vi "Item Selection VIG - Originale.vi"(4 "Defer Front Panel (T)":bool, 6 "Shift":bool, 7 "Method (Read Selection)":T1, 8 "error in (no error)":errorcluster, 9 "New Selected Row":i32, 10 "Selection":bool[](array[boolean]), 11 "Listbox or Tree":refnum<vi>) -> (0 "error out":errorcluster, 2 "Tags":string[](array[string]), 3 "Selection":bool[](array[boolean]))   [LabVIEW 2020]
doc: "This is a global VI that maintains the state of <B>Listbox</B> passed in. The first this this is called it should have the <B>Method</B> set to Force Selection which sets the symbols of the contol based on <B>Selection</B>. This VI can then be called to select all, select none, or invert the selection of that control. This VI can also handle the mouse down event on the control, which will set or clear the selection of items based on the <B>New Selected Row</B>, and if the <B>Shift</B> key was being held. The default method will return the <B>Selected Items</B> for that control.\n\nBy default this VI will <B>Defer Front Panel</B> of the front panel of the owning VI and undefer after the selection has finished.\n-------------\nBrian Hoover (hooovahh)"
uses:
  Selection Global Method.ctl
  <userlib>/_OpenG.lib/array/array.llb/Conditional Auto-Indexing Tunnel (String)__ogtk.vi
  <userlib>/_OpenG.lib/array/array.llb/Search 1D Array (Boolean)__ogtk.vi
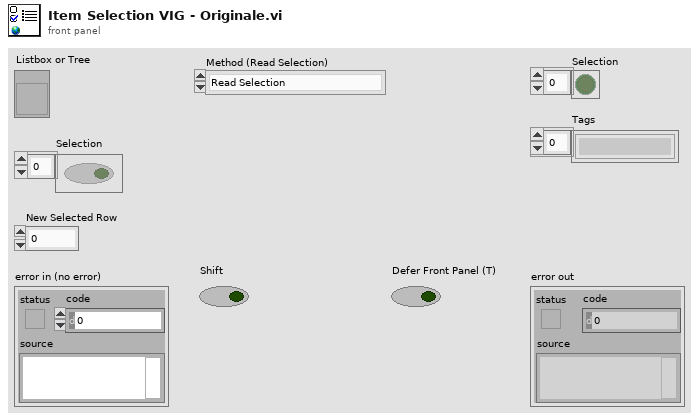
[diagram p1: front panel]
types:
  T1 = typedef "Selection Global Method.ctl" = enum16{"Read Selection", "Force Selection", "Mouse Down Event", "Select All", "Select None", "Invert Selection", "Read Selection and Tags"}
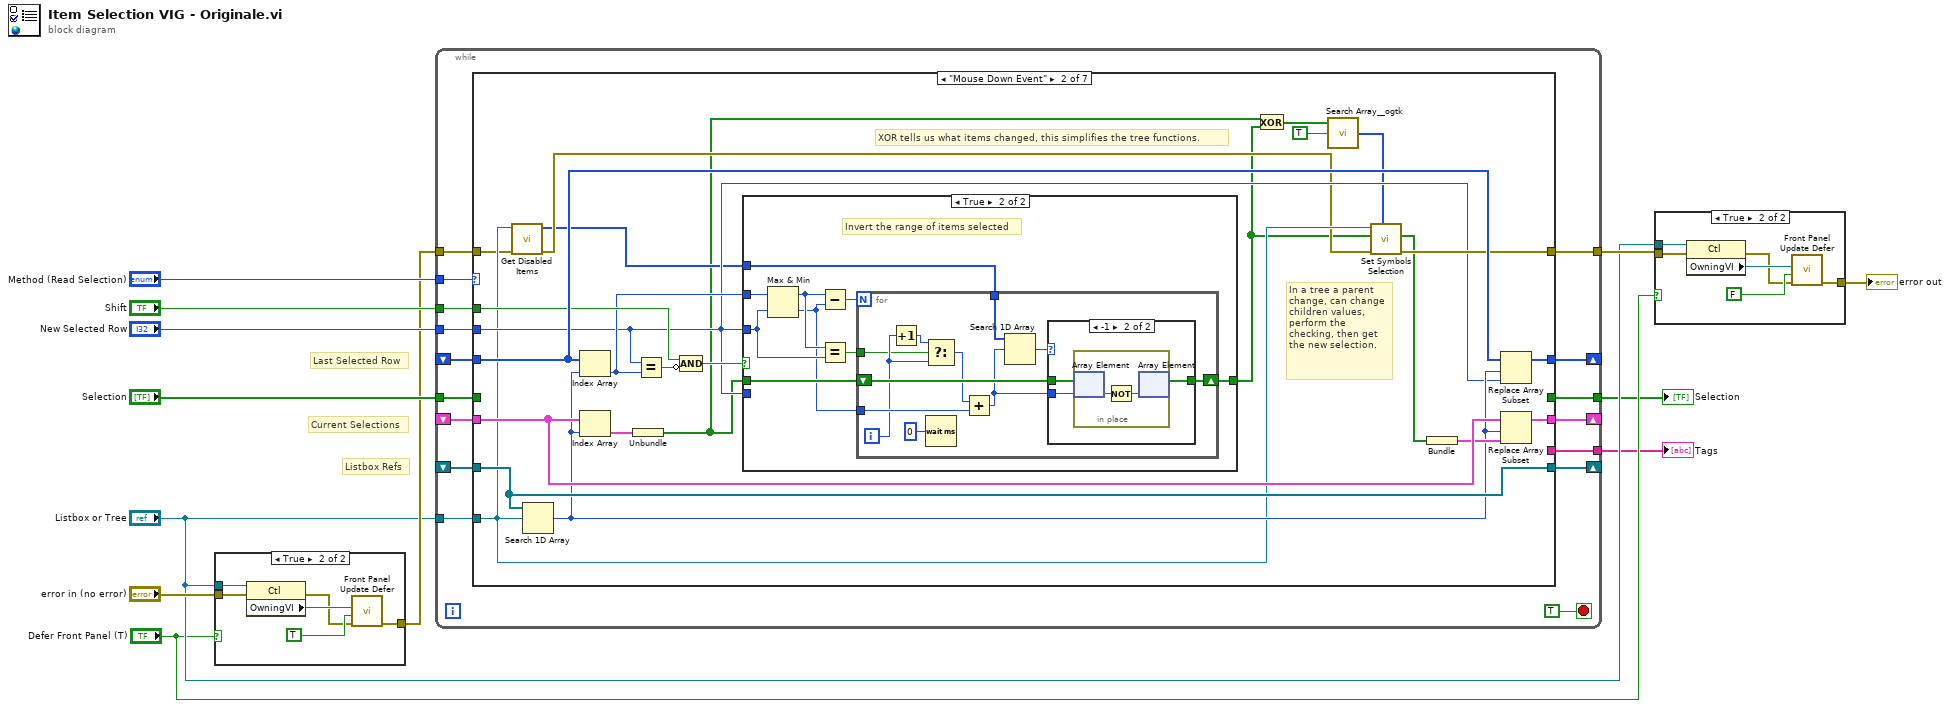
[diagram p0: block diagram]
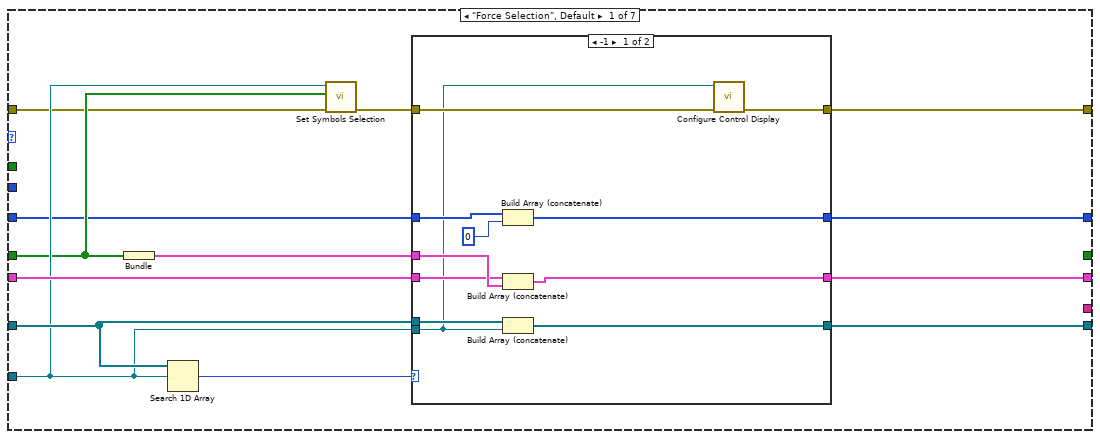
[diagram p4: hidden frame]
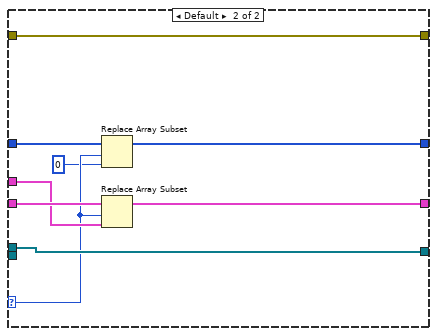
[diagram p5: hidden frame]
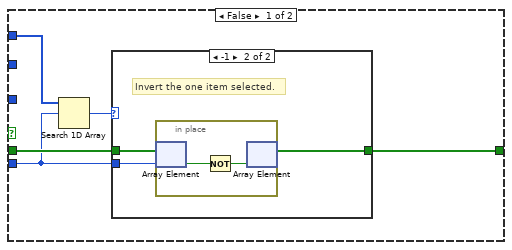
[diagram p6: hidden frame]
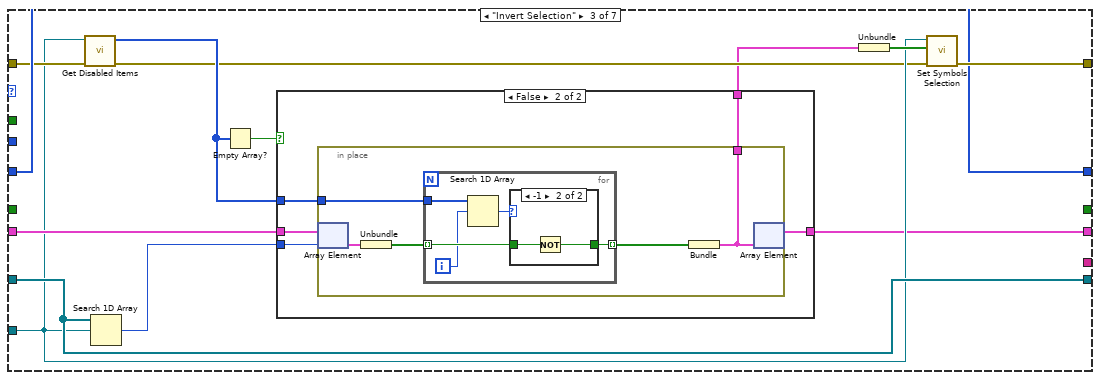
[diagram p9: hidden frame]
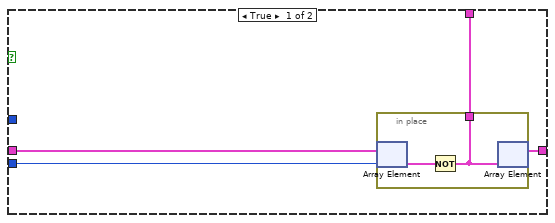
[diagram p10: hidden frame]
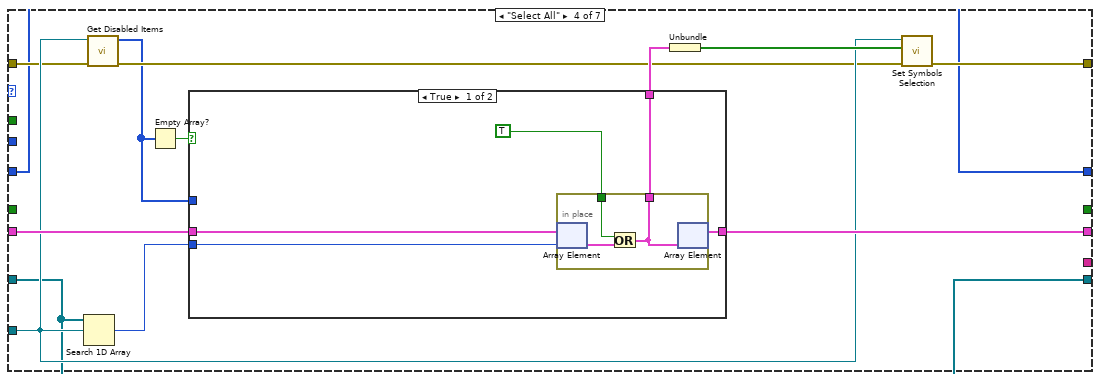
[diagram p12: hidden frame]
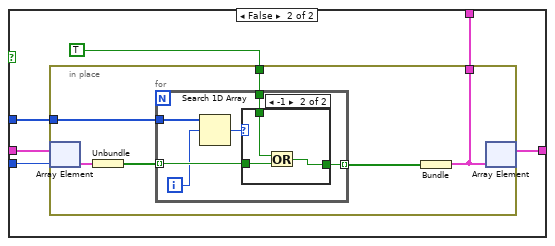
[diagram p13: hidden frame]
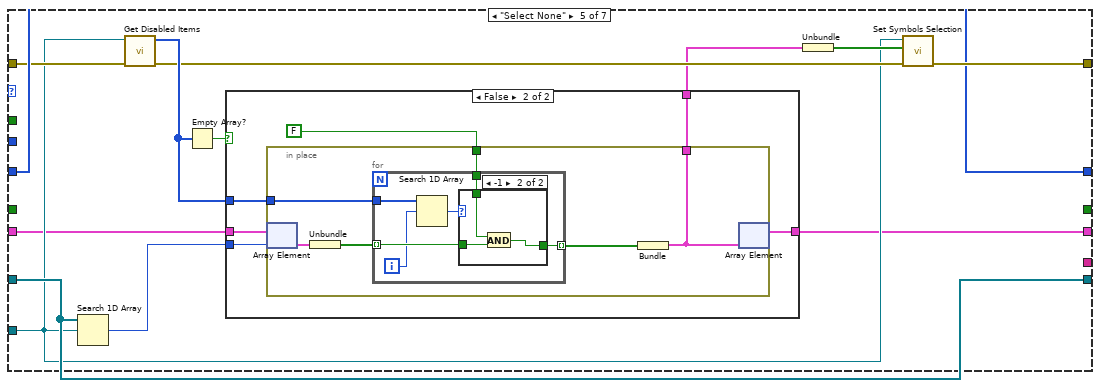
[diagram p15: hidden frame]
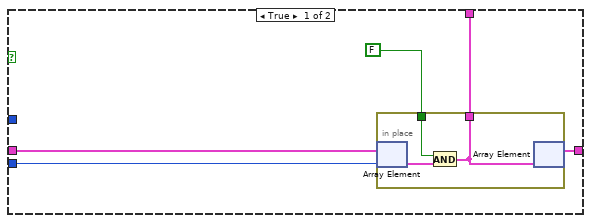
[diagram p16: hidden frame]
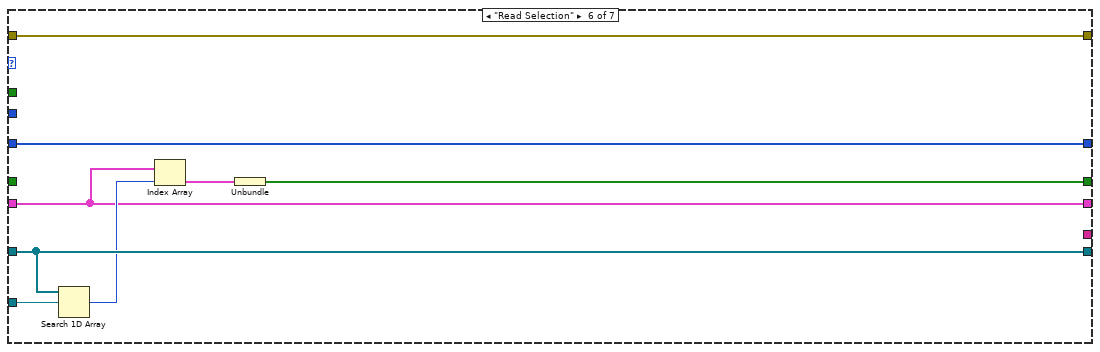
[diagram p18: hidden frame]
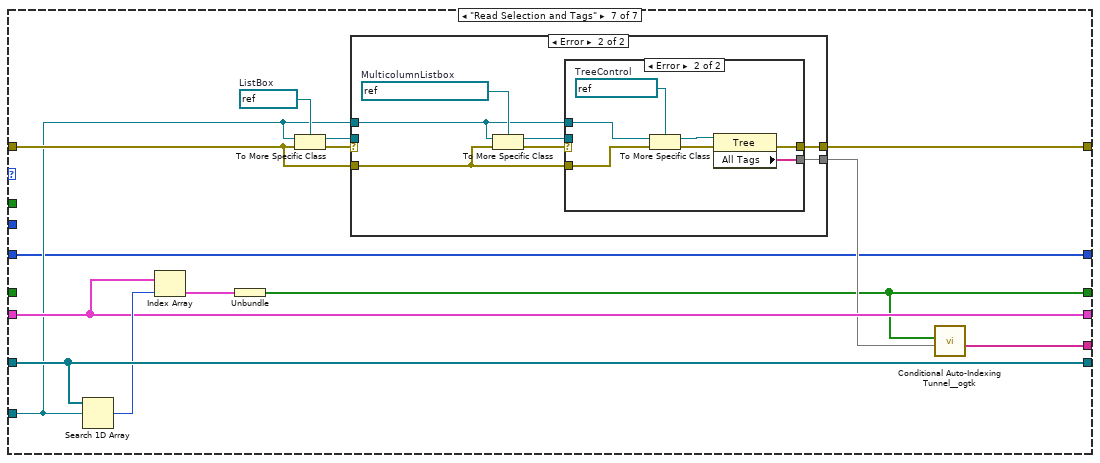
[diagram p19: hidden frame]
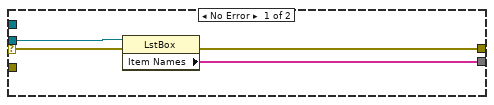
[diagram p20: hidden frame]
diagram:
  # "Listbox Refs"
  # "Current Selections"
  # "Last Selected Row"
  n1 = case shown="True" "Defer Front Panel (T)" {
    tunnel: "Listbox or Tree" -> [_ w19]
    tunnel: "error in (no error)" -> [w13 w15]
    tunnel: [w13 w14] -> w7
    frame False {
    }
    frame True {
      n2 = property class="Ctl"(reference=w19, error in=w15) -> (error out=w16:errorcluster, "OwningVI"=w18:refnum<vi>)  [unwired: 1 out]
      n3 = call "Front Panel Update Defer.vi"("error in (no error)"=w16, "Defer Panel Updates? (F)"=TRUE, "VI Reference (Calling VI)"=w18) -> ("error out"=w14:errorcluster)  [unwired: 8 in]
    }
  }
  n4 = while {
    tunnel: "Method (Read Selection)" -> [w35]
    tunnel: "Listbox or Tree" -> [w33]
    shift-right: [w32] -> _
    shift-left: _ -> [w31]
    tunnel: "Selection" -> [w30]
    shift-right: [w29] -> _
    shift-left: _ -> [w28]
    tunnel: w7 -> [w27]
    shift-right: [w26] -> _
    shift-left: _ -> [w25]
    tunnel: "New Selected Row" -> [w24]
    tunnel: "Shift" -> [w23]
    tunnel: [w22] -> w6
    tunnel: [w21] -> w2
    tunnel: [w20] -> w1
    stop <- TRUE stop-if-true
    n5 = case shown="\"Mouse Down Event\"" w35 {
      tunnel: w33 -> [w42 w78 w133 w173 w215 w260 w265]
      tunnel: [w47 w83 w140 w168 w219 w259 w274] -> w32
      tunnel: w31 -> [w46 w83 w140 w168 w219 w259 w274]
      tunnel: w30 -> [w41 _ _ _ _ _ _]
      tunnel: [w44 w88 w131 w175 w210 w255 w272] -> w29
      tunnel: w28 -> [w43 w92 w136 w179 w213 w255 w272]
      tunnel: w27 -> [w40 w77 w134 w172 w217 w257 w267]
      tunnel: [w39 w89 w139 w169 w220 w258 w261] -> w26
      tunnel: w25 -> [w38 w90 w139 w169 w220 w258 w261]
      tunnel: w24 -> [_ w79 _ _ _ _ _]
      tunnel: w23 -> [_ w87 _ _ _ _ _]
      tunnel: [w36 w81 w141 w174 w221 w257 w266] -> w22
      tunnel: [_ _ _ _ _ w253 w263] -> w21
      tunnel: [_ _ _ _ _ _ w262] -> w20
      frame "Force Selection", Default {
        n6 = Bundle("Selection"=w41) -> (w45:cluster{"Selection":bool[]})  [unwired: 1 in]
        n7 = Search 1D Array(1D array=w46, element=w42) -> (index of element=w48:i32)  [unwired: 1 in]
        n8 = call "Set Symbols Selection.vi"("error in (no error)"=w40, "Selected Items In"=w41, "Listbox or Tree"=w42) -> ("error out"=w37:errorcluster)  [unwired: 7 in, 1 out]
        n9 = case shown="-1" w48 {
          selector: w48 -> [_ w62]
          tunnel: w42 -> [w50 _]
          tunnel: [w59 w68] -> w47
          tunnel: w46 -> [w58 w68]
          tunnel: w45 -> [w57 w65]
          tunnel: [w56 w66] -> w44
          tunnel: w43 -> [w55 w67]
          tunnel: [w53 w63] -> w39
          tunnel: w38 -> [w52 w64]
          tunnel: w37 -> [w51 w60]
          tunnel: [w49 w60] -> w36
          frame -1 {
            n10 = Build Array (concatenate)(w52, 0) -> (w53:i32[])
            n11 = Build Array (concatenate)(w55, w57) -> (w56:cluster{"Selection":bool[]}[])
            n12 = Build Array (concatenate)(w58, w50) -> (w59:refnum<vi>[])
            n13 = call "Configure Control Display.vi"("error in (no error)"=w51, "Listbox or Tree"=w50) -> ("error out"=w49:errorcluster)  [unwired: 9 in]
          }
          frame Default {
            n14 = Replace Array Subset(array=w64, new element=0, index=w62) -> (w63:i32[])
            n15 = Replace Array Subset(array=w67, new element=w65, index=w62) -> (w66:cluster{"Selection":bool[]}[])
          }
        }
      }
      frame "Mouse Down Event" {
        # "In a tree a parent change, can change children values, perform the checking, then get the new selection."
        # "XOR tells us what items changed, this simplifies the tree functions."
        n16 = call "Get Disabled Items.vi"("error in (no error)"=w77, "Listbox or Tree"=w78) -> ("error out"=w76:errorcluster, "Disabled Items"=w75:i32[])  [unwired: 8 in]
        n17 = Search 1D Array(1D array=w83, element=w78) -> (index of element=w80:i32)  [unwired: 1 in]
        n18 = Index Array(array=w90, index=w80) -> (element=w82:i32)
        n19 = Index Array(array=w92, index=w80) -> (element=w91:cluster{"Selection":bool[]})
        n20 = Unbundle(w91) -> ("Selection"=w73:bool[])
        n21 = Equal?(x=w79, y=w82) -> (x = y?=w86:bool)
        n22 = Compound Arithmetic op=AND(w87, invert w86) -> (w84:bool)
        n23 = case shown="True" w84 {
          tunnel: w73 -> [w97 w108]
          tunnel: w79 -> [w94 _]
          tunnel: [w96 w107] -> w74
          tunnel: w79 -> [_ w111]
          tunnel: w82 -> [_ w112]
          tunnel: w75 -> [w95 w104]
          frame False {
            n24 = Search 1D Array(1D array=w95, element=w94) -> (index of element=w93:i32)  [unwired: 1 in]
            n25 = case shown="-1" w93 {
              tunnel: w97 -> [w98 w101]
              tunnel: [w98 w100] -> w96
              tunnel: w94 -> [_ w99]
              frame Default {
              }
              frame -1 {
                # "Invert the one item selected."
                n26 = in-place {
                  n27 = in-place-array #1(w101, w99) -> (w103:bool)
                  n28 = Not(x=w103) -> (.not. x?=w102:bool)
                  n29 = in-place-array #1(w102) -> (w100:bool[])  [unwired: 1 out]
                }
              }
            }
          }
          frame True {
            # "Invert the range of items selected"
            n30 = Max & Min(x=w112, y=w111) -> (max(x,y)=w110:i32, min(x,y)=w106:i32)
            n31 = Subtract(x=w110, y=w106) -> (x-y=w109:i32)
            n32 = Equal?(x=w110, y=w111) -> (x = y?=w105:bool)
            n33 = for {
              N: w109 -> [_]
              shift-right: [w122] -> w107
              shift-left: w108 -> [w123]
              tunnel: w106 -> [w121]
              tunnel: w105 -> [w117]
              tunnel: w104 -> [w115]
              i -> [w119]
              n34 = Increment(x=w119) -> (x+1=w118:i32)
              n35 = Select(t=w118, s=w117, f=w119) -> (s? t:f=w120:i32)
              n36 = Wait (ms)(milliseconds to wait=u32 0) -> ()  [unwired: 1 out]
              n37 = Add(x=w120, y=w121) -> (x+y=w114:i32)
              n38 = Search 1D Array(1D array=w115, element=w114) -> (index of element=w113:i32)  [unwired: 1 in]
              n39 = case shown="-1" w113 {
                tunnel: w123 -> [w124 w127]
                tunnel: [w124 w126] -> w122
                tunnel: w114 -> [_ w125]
                frame Default {
                }
                frame -1 {
                  n40 = in-place {
                    n41 = in-place-array #2(w127, w125) -> (w129:bool)
                    n42 = Not(x=w129) -> (.not. x?=w128:bool)
                    n43 = in-place-array #2(w128) -> (w126:bool[])  [unwired: 1 out]
                  }
                }
              }
            }
          }
        }
        n44 = Exclusive Or(1:w74, 2:w73) -> (0:w72:bool[])
        n45 = call-poly <userlib>:"Search Array__ogtk.vi"("Array"=w72, "Element Data"=TRUE) -> ("Indices of Elements"=w70:i32[])  [unwired: 7 in]
        n46 = call "Set Symbols Selection.vi"("Indices Modified"=w70, "error in (no error)"=w76, "Selected Items In"=w74, "Listbox or Tree"=w78) -> ("error out"=w81:errorcluster, "Selected Items Out"=w69:bool[])  [unwired: 6 in]
        n47 = Bundle("Selected Items Out"=w69) -> (w85:cluster{"Selected Items Out":bool[]})  [unwired: 1 in]
        n48 = Replace Array Subset(array=w90, new element=w79, index=w80) -> (w89:i32[])
        n49 = Replace Array Subset(array=w92, new element=w85, index=w80) -> (w88:cluster{"Selection":bool[]}[])
      }
      frame "Invert Selection" {
        n50 = call "Get Disabled Items.vi"("error in (no error)"=w134, "Listbox or Tree"=w133) -> ("error out"=w132:errorcluster, "Disabled Items"=w137:i32[])  [unwired: 8 in]
        n51 = Search 1D Array(1D array=w140, element=w133) -> (index of element=w135:i32)  [unwired: 1 in]
        n52 = Empty Array?(array=w137) -> (empty?=w138:bool)
        n53 = case shown="False" w138 {
          tunnel: w136 -> [w146 w153]
          tunnel: w135 -> [w145 w152]
          tunnel: [w144 w151] -> w130
          tunnel: [w143 w150] -> w131
          tunnel: w137 -> [_ w149]
          frame True {
            n54 = in-place {
              in-place-border: [w147] -> w144
              n55 = in-place-array #3(w146, w145) -> (w148:cluster{"Selection":bool[]})
              n56 = Not(x=w148) -> (.not. x?=w147:cluster{"Selection":bool[]})
              n57 = in-place-array #3(w147) -> (w143:cluster{"Selection":bool[]}[])  [unwired: 1 out]
            }
          }
          frame False {
            n58 = in-place {
              in-place-border: [w154] -> w151
              in-place-border: w149 -> [w156]
              n59 = in-place-array #4(w153, w152) -> (w158:cluster{"Selection":bool[]})
              n60 = Unbundle(w158) -> ("Selection"=w157:bool[])
              n61 = for {
                tunnel: w157 -> [w163] mode=indexing
                tunnel: w156 -> [w162]
                tunnel: [w159] -> w155 mode=indexing
                i -> [w161]
                n62 = Search 1D Array(1D array=w162, element=w161) -> (index of element=w160:i32)  [unwired: 1 in]
                n63 = case shown="-1" w160 {
                  tunnel: w163 -> [w164 w166]
                  tunnel: [w164 w165] -> w159
                  frame Default {
                  }
                  frame -1 {
                    n64 = Not(x=w166) -> (.not. x?=w165:bool)
                  }
                }
              }
              n65 = Bundle(w155) -> (w154:cluster{bool[]})  [unwired: 1 in]
              n66 = in-place-array #4(w154) -> (w150:cluster{"Selection":bool[]}[])  [unwired: 1 out]
            }
          }
        }
        n67 = Unbundle(w130) -> ("Selection"=w142:bool[])
        n68 = call "Set Symbols Selection.vi"("error in (no error)"=w132, "Selected Items In"=w142, "Listbox or Tree"=w133) -> ("error out"=w141:errorcluster)  [unwired: 7 in, 1 out]
      }
      frame "Select All" {
        n69 = Search 1D Array(1D array=w168, element=w173) -> (index of element=w178:i32)  [unwired: 1 in]
        n70 = call "Get Disabled Items.vi"("error in (no error)"=w172, "Listbox or Tree"=w173) -> ("error out"=w171:errorcluster, "Disabled Items"=w167:i32[])  [unwired: 8 in]
        n71 = Empty Array?(array=w167) -> (empty?=w170:bool)
        n72 = case shown="True" w170 {
          tunnel: w179 -> [w184 w193]
          tunnel: w178 -> [w183 w192]
          tunnel: [w182 w191] -> w177
          tunnel: [w181 w190] -> w175
          tunnel: w167 -> [_ w188]
          frame True {
            n73 = in-place {
              in-place-border: [w186] -> w182
              in-place-border: TRUE ("Boolean") -> [w185]
              n74 = in-place-array #5(w184, w183) -> (w187:cluster{"Selection":bool[]})
              n75 = Or(x=w185, y=w187) -> (x .or. y?=w186:cluster{"Selection":bool[]})
              n76 = in-place-array #5(w186) -> (w181:cluster{"Selection":bool[]}[])  [unwired: 1 out]
            }
          }
          frame False {
            n77 = in-place {
              in-place-border: [w194] -> w191
              in-place-border: TRUE ("Boolean") -> [w197]
              in-place-border: w188 -> [w196]
              n78 = in-place-array #6(w193, w192) -> (w199:cluster{"Selection":bool[]})
              n79 = Unbundle(w199) -> ("Selection"=w198:bool[])
              n80 = for {
                tunnel: w198 -> [w204] mode=indexing
                tunnel: w197 -> [w205]
                tunnel: w196 -> [w203]
                tunnel: [w200] -> w195 mode=indexing
                i -> [w202]
                n81 = Search 1D Array(1D array=w203, element=w202) -> (index of element=w201:i32)  [unwired: 1 in]
                n82 = case shown="-1" w201 {
                  tunnel: w205 -> [_ w209]
                  tunnel: w204 -> [w206 w208]
                  tunnel: [w206 w207] -> w200
                  frame Default {
                  }
                  frame -1 {
                    n83 = Or(x=w209, y=w208) -> (x .or. y?=w207:bool)
                  }
                }
              }
              n84 = Bundle(w195) -> (w194:cluster{bool[]})  [unwired: 1 in]
              n85 = in-place-array #6(w194) -> (w190:cluster{"Selection":bool[]}[])  [unwired: 1 out]
            }
          }
        }
        n86 = Unbundle(w177) -> ("Selection"=w176:bool[])
        n87 = call "Set Symbols Selection.vi"("error in (no error)"=w171, "Selected Items In"=w176, "Listbox or Tree"=w173) -> ("error out"=w174:errorcluster)  [unwired: 7 in, 1 out]
      }
      frame "Select None" {
        n88 = Search 1D Array(1D array=w219, element=w215) -> (index of element=w214:i32)  [unwired: 1 in]
        n89 = call "Get Disabled Items.vi"("error in (no error)"=w217, "Listbox or Tree"=w215) -> ("error out"=w216:errorcluster, "Disabled Items"=w218:i32[])  [unwired: 8 in]
        n90 = Empty Array?(array=w218) -> (empty?=w212:bool)
        n91 = case shown="False" w212 {
          tunnel: w213 -> [w227 w236]
          tunnel: w214 -> [w226 w235]
          tunnel: [w225 w234] -> w211
          tunnel: [w224 w233] -> w210
          tunnel: w218 -> [_ w231]
          frame True {
            n92 = in-place {
              in-place-border: [w229] -> w225
              in-place-border: FALSE ("Boolean") -> [w228]
              n93 = in-place-array #7(w227, w226) -> (w230:cluster{"Selection":bool[]})
              n94 = And(x=w228, y=w230) -> (x .and. y?=w229:cluster{"Selection":bool[]})
              n95 = in-place-array #7(w229) -> (w224:cluster{"Selection":bool[]}[])  [unwired: 1 out]
            }
          }
          frame False {
            n96 = in-place {
              in-place-border: [w237] -> w234
              in-place-border: FALSE ("Boolean") -> [w240]
              in-place-border: w231 -> [w239]
              n97 = in-place-array #8(w236, w235) -> (w242:cluster{"Selection":bool[]})
              n98 = Unbundle(w242) -> ("Selection"=w241:bool[])
              n99 = for {
                tunnel: w241 -> [w247] mode=indexing
                tunnel: w240 -> [w248]
                tunnel: w239 -> [w246]
                tunnel: [w243] -> w238 mode=indexing
                i -> [w245]
                n100 = Search 1D Array(1D array=w246, element=w245) -> (index of element=w244:i32)  [unwired: 1 in]
                n101 = case shown="-1" w244 {
                  tunnel: w248 -> [_ w252]
                  tunnel: w247 -> [w249 w251]
                  tunnel: [w249 w250] -> w243
                  frame Default {
                  }
                  frame -1 {
                    n102 = And(x=w252, y=w251) -> (x .and. y?=w250:bool)
                  }
                }
              }
              n103 = Bundle(w238) -> (w237:cluster{bool[]})  [unwired: 1 in]
              n104 = in-place-array #8(w237) -> (w233:cluster{"Selection":bool[]}[])  [unwired: 1 out]
            }
          }
        }
        n105 = Unbundle(w211) -> ("Selection"=w222:bool[])
        n106 = call "Set Symbols Selection.vi"("error in (no error)"=w216, "Selected Items In"=w222, "Listbox or Tree"=w215) -> ("error out"=w221:errorcluster)  [unwired: 7 in, 1 out]
      }
      frame "Read Selection" {
        n107 = Search 1D Array(1D array=w259, element=w260) -> (index of element=w256:i32)  [unwired: 1 in]
        n108 = Index Array(array=w255, index=w256) -> (element=w254:cluster{"Selection":bool[]})
        n109 = Unbundle(w254) -> ("Selection"=w253:bool[])
      }
      frame "Read Selection and Tags" {
        w270 = refnum<vi> refnum  # ListBox
        n110 = Search 1D Array(1D array=w274, element=w265) -> (index of element=w273:i32)  [unwired: 1 in]
        n111 = Index Array(array=w272, index=w273) -> (element=w271:cluster{"Selection":bool[]})
        n112 = Unbundle(w271) -> ("Selection"=w263:bool[])
        n113 = To More Specific Class(target class=w270, reference=w265, error in=w267) -> (specific class reference=w268:refnum<vi>, error out=w269:errorcluster)
        n114 = case shown="Error" w269 {
          selector: w269 -> [w277 _]
          tunnel: w268 -> [w278 _]
          tunnel: w267 -> [_ w281]
          tunnel: [w276 w282] -> w266
          tunnel: w265 -> [_ w280]
          tunnel: [w275 w279] -> w264
          frame No Error {
            n115 = property class="LstBox"(reference=w278, error in=w277) -> (error out=w276:errorcluster, "Item Names"=w275:string[])  [unwired: 1 out]
          }
          frame Error {
            w285 = refnum<vi> refnum  # MulticolumnListbox
            n116 = To More Specific Class(target class=w285, reference=w280, error in=w281) -> (specific class reference=w284:refnum<vi>, error out=w283:errorcluster)
            n117 = case shown="Error" w283 {
              selector: w283 -> [w289 _]
              tunnel: [w291 w292] -> w282
              tunnel: w284 -> [w290 _]
              tunnel: w281 -> [_ w297]
              tunnel: w280 -> [_ w296]
              tunnel: [w286 w294] -> w279
              frame No Error {
                n118 = property class="MCListbox"(reference=w290, error in=w289) -> (error out=w291:errorcluster, "ItemNames"=w287:string[][])  [unwired: 1 out]
                n119 = Index Array(array=w287, index (col)=0 ("disabled index (col)")) -> (element=w286:string[])  [unwired: 1 in]
              }
              frame Error {
                w298 = refnum<vi> refnum  # TreeControl
                n120 = To More Specific Class(target class=w298, reference=w296, error in=w297) -> (specific class reference=w295:refnum<vi>, error out=w293:errorcluster)
                n121 = property class="Tree"(reference=w295, error in=w293) -> (error out=w292:errorcluster, "All Tags"=w294:string[])  [unwired: 1 out]
              }
            }
          }
        }
        n122 = call-poly <userlib>:"Conditional Auto-Indexing Tunnel__ogtk.vi"("Array in"=w264, "Elements to keep"=w263) -> ("Filtered Array out"=w262:string[])  [unwired: 5 in]
      }
    }
  }
  "Selection" <- w2
  "Tags" <- w1
  n123 = case shown="True" "Defer Front Panel (T)" {
    tunnel: "Listbox or Tree" -> [_ w305]
    tunnel: w6 -> [w299 w301]
    tunnel: [w299 w300] -> w3
    frame False {
    }
    frame True {
      n124 = property class="Ctl"(reference=w305, error in=w301) -> (error out=w302:errorcluster, "OwningVI"=w304:refnum<vi>)  [unwired: 1 out]
      n125 = call "Front Panel Update Defer.vi"("error in (no error)"=w302, "Defer Panel Updates? (F)"=FALSE, "VI Reference (Calling VI)"=w304) -> ("error out"=w300:errorcluster)  [unwired: 8 in]
    }
  }
  "error out" <- w3
